vi "ALS Feedback DO ref.vi"(10 "DAQ ref.AO ref":refnum<vi>[](array[refnum]), 11 "DAQ ref.DO ref":refnum<vi>[](array[refnum])) -> ()   [LabVIEW 2022 SP3]
uses:
  Sub VI's/Global 1.vi
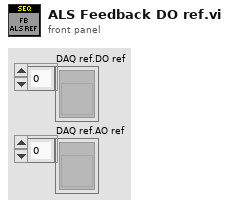
[diagram p1: front panel]
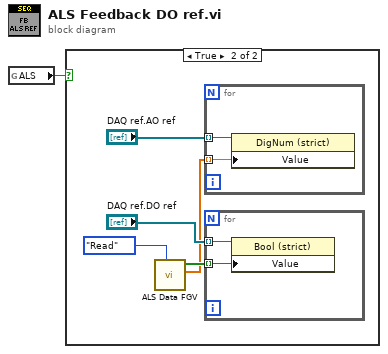
[diagram p0: block diagram]
diagram:
  n1 = global read "Global 1.vi" "ALS"() -> (w1:bool)
  n2 = case shown="True" w1 {
    frame False {
    }
    frame True {
      n3 = call "ALS Data FGV.vi"("Enum"=enum16{"Read", "Write"}."Read") -> ("ALS AO out"=w3:dbl[], "ALS DO out"=w5:bool[])  [unwired: 8 in, 1 out]
      n4 = for {
        tunnel: "DAQ ref.AO ref" -> [w8] mode=indexing
        tunnel: w3 -> [w7] mode=indexing
        n5 = property class="DigNum (strict)"(reference=w8, "Value"=w7) -> ()  [unwired: 1 in, 2 out]
      }
      n6 = for {
        tunnel: "DAQ ref.DO ref" -> [w10] mode=indexing
        tunnel: w5 -> [w9] mode=indexing
        n7 = property class="Bool (strict)"(reference=w10, "Value"=w9) -> ()  [unwired: 1 in, 2 out]
      }
    }
  }
